vi "Hand_auto_switch.vi"(2 "t_reset":u32=1000, 3 "Hand":bool, 4 "Auto":bool) -> (0 "reset":bool, 1 "Z1":u32)   [LabVIEW 2019, in "Logik.lvlib"]
uses:
  Logik.lvlib
  fronts.vi
  Trigers/RS.vi
  Timer Delay/Timers.lvlib
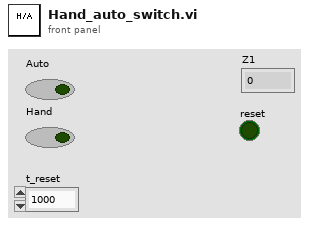
[diagram p1: front panel]
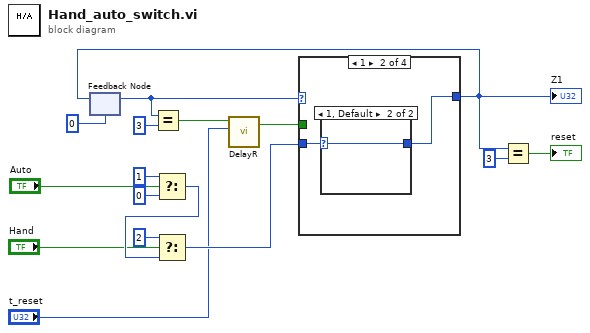
[diagram p0: block diagram]
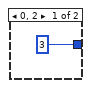
[diagram p3: hidden frame]
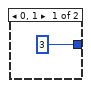
[diagram p5: hidden frame]
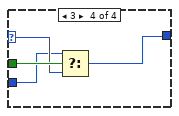
[diagram p6: hidden frame]
diagram:
  n1 = feedback #1(u32 0) -> (w8:u32)
  n2 = Equal?(x=w8, y=u32 3) -> (x = y?=w3:bool)
  n3 = Select(t=u32 1, s="Auto", f=u32 0) -> (s? t:f=w14:u32)
  n4 = Select(t=u32 2, s="Hand", f=w14) -> (s? t:f=w10:u32)
  n5 = call "DelayR.vi"("DelayOn"="t_reset", "In"=w3) -> ("Out"=w1:bool)  [unwired: 2 in, 1 out]
  n6 = case shown="1" w8 {
    selector: w8 -> [_ _ _ w28]
    tunnel: [w17 w18 w23 w26] -> w5
    tunnel: w10 -> [w17 w19 w22 w27]
    tunnel: w1 -> [_ _ _ w29]
    frame 0, Default {
    }
    frame 1 {
      n7 = case shown="1, Default" w19 {
        selector: w19 -> [_ w21]
        tunnel: [u32 3 w21] -> w18
        frame 0, 2 {
        }
        frame 1, Default {
        }
      }
    }
    frame 2 {
      n8 = case shown="2, Default" w22 {
        selector: w22 -> [_ w25]
        tunnel: [u32 3 w25] -> w23
        frame 0, 1 {
        }
        frame 2, Default {
        }
      }
    }
    frame 3 {
      n9 = Select(t=w27, s=w29, f=w28) -> (s? t:f=w26:u32)
    }
  }
  "Z1" <- w5
  n10 = feedback-in #1(w5) -> ()
  n11 = Equal?(x=w5, y=u32 3) -> (x = y?=→"reset":bool)
